vi "lib create TID folder.vi"(8 "error in (no error)":errorcluster, 10 "Root":path, 11 "TID Info":T1) -> (0 "error out":errorcluster, 2 "TID Name":string, 3 "TID Folder":path)   [LabVIEW 2011]
uses:
  DownSample/typedefs/Downsample TID Info cluster.ctl
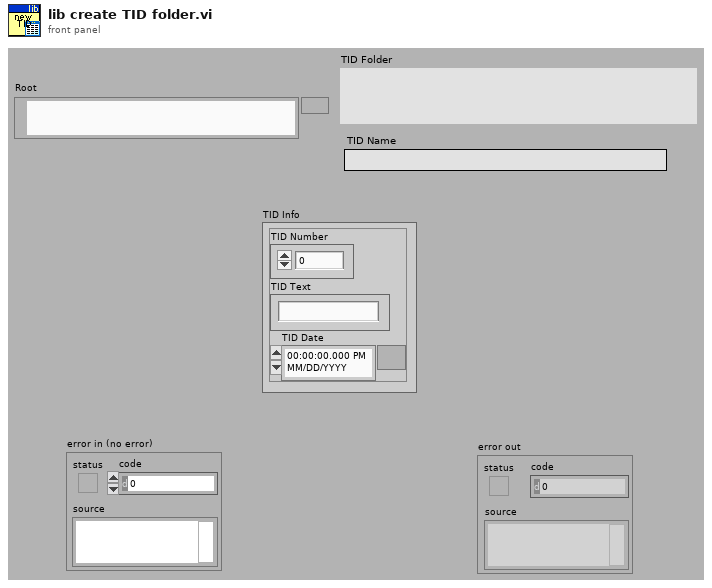
[diagram p1: front panel]
types:
  T1 = typedef "Downsample TID Info cluster.ctl" = cluster{"TID Number":u32, "TID Text":string, "TID Date":timestamp}
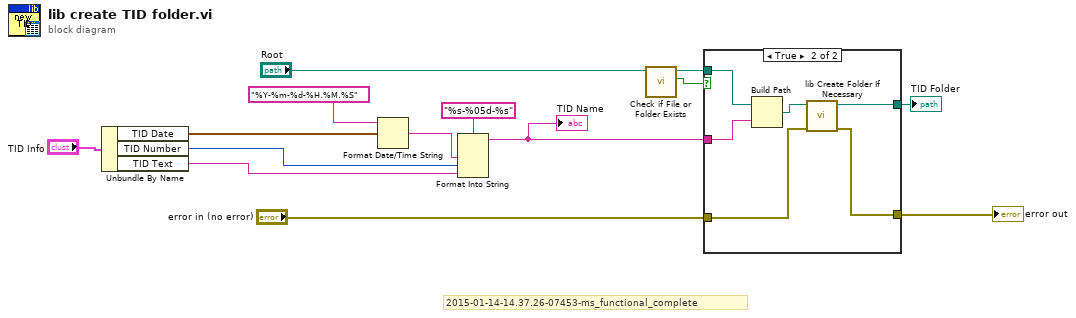
[diagram p0: block diagram]
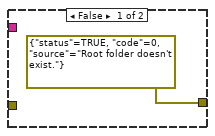
[diagram p2: hidden frame]
diagram:
  # "2015-01-14-14.37.26-07453-ms_functional_complete"
  n1 = Unbundle By Name("TID Info") -> ("TID Date"=w3:timestamp, "TID Number"=w2:u32, "TID Text"=w1:string)
  n2 = Format Date/Time String(time format string (%c)="%Y-%m-%d-%H.%M.%S", seconds (now)=w3) -> (date/time string=w12:string)  [unwired: 1 in]
  n3 = Format Into String(format string="%s-%05d-%s", w12, w2, w1) -> (resulting string=w8:string)  [unwired: 2 in, 1 out]
  "TID Name" <- w8
  n4 = call <vilib>:"Check if File or Folder Exists.vi"("path"="Root") -> ("file or folder exists?"=w9:bool, "dup path"=w10:path)  [unwired: 8 in, 1 out]
  n5 = case shown="True" w9 {
    tunnel: w10 -> [_ w21]
    tunnel: w8 -> [_ w20]
    tunnel: "error in (no error)" -> [_ w18]
    tunnel: [errorcluster {"status"=TRUE, "code"=0, "source"="Root folder doesn't exist."} ("error out") w17] -> w6
    tunnel: [_ w16] -> w5
    frame False {
    }
    frame True {
      n6 = Build Path(base path=w21, name or relative path=w20) -> (appended path=w19:path)
      n7 = call "lib Create Folder If Necessary.vi"("error in (no error)"=w18, "Folder"=w19) -> ("error out"=w17:errorcluster, "Folder dup"=w16:path)  [unwired: 8 in]
    }
  }
  "error out" <- w6
  "TID Folder" <- w5
